vi "Формула Проницаемости.vi"(10 "Р атм..":dbl format="%#.3g", 11 "P пластовое":dbl format="%#.3g") -> (0 "Давление по пересчету":dbl format="%#.2g")   [LabVIEW 2018]
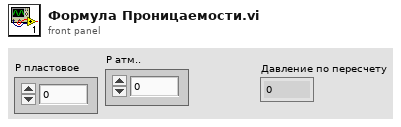
[diagram p1: front panel]
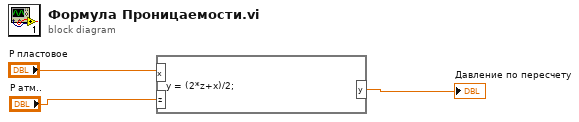
[diagram p0: block diagram]
diagram:
  n1 = formula code="y = (2*z+x)/2;"("x"="P пластовое", "z"="Р атм..") -> ("y"=→"Давление по пересчету":dbl)
